vi "Untitled 2.vi"() -> ()   [LabVIEW 2017]
uses:
  <vilib>/Rock Robotics/SystemInterfaces/DIO/FPGA_DIOPWMChannel.ctl
  <vilib>/Rock Robotics/WPI/Joystick/WPI_JoystickDeviceEnum.ctl
  <vilib>/Rock Robotics/WPI/MotorControl/WPI_MotorControlOpen TalonSRX.vi
panel:
  in  "Output":dbl
  in  "stop":bool
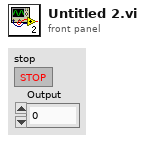
[diagram p1: front panel]
types:
  T1 = typedef "WPI_JoystickDeviceEnum.ctl" = enum16{"USB 0", "USB 1", "USB 2", "USB 3", "USB 4", "USB 5"}
  T2 = typedef "FPGA_DIOPWMChannel.ctl" = enum8{"PWM 0", "PWM 1", "PWM 2", "PWM 3", "PWM 4", "PWM 5", "PWM 6", "PWM 7", "PWM 8", "PWM 9", "PWM MXP 0", "PWM MXP 1", "PWM MXP 2", "PWM MXP 3", "PWM MXP 4", "PWM MXP 5", "PWM MXP 6", "PWM MXP 7", "PWM MXP 8", "PWM MXP 9", "Invalid"}
  T3 = typedef "WPI_MotorControlDeviceRef.ctl" = cluster{"DeviceStatus":errorcluster, "Type":T4, "PWM":cluster{"PWM Channel":T2, "DeadBand":T5}, "CAN":cluster{"Device Number":u8, "SetOutput VI Ref":variant, "GetOutput VI Ref":variant, "Enable VI Ref":variant, "Disable VI Ref":variant, "Data":variant}, "Invert":bool, "DIO PWM":cluster{"PWM \"Enable\" Channel":T2, "DIOChannel":T6, "PWM Rate":dbl}}
  T4 = typedef "WPI_MotorControlType.ctl" = enum16{"PWM", "CAN", "DIO PWM"}
  T5 = typedef "WPI_PWMDeadband.ctl" = cluster{"Name":string, "maxPositivePwm":i32, "minPositivePwm":i32, "centerPwm":i32, "maxNegativePwm":i32, "minNegativePwm":i32, "angularRange":u16}
  T6 = typedef "FPGA_DIOChannel.ctl" = enum8{"DIO 0", "DIO 1", "DIO 2", "DIO 3", "DIO 4", "DIO 5", "DIO 6", "DIO 7", "DIO 8", "DIO 9", "DIO MXP 0", "DIO MXP 1", "DIO MXP 2", "DIO MXP 3", "DIO MXP 4", "DIO MXP 5", "DIO MXP 6", "DIO MXP 7", "DIO MXP 8", "DIO MXP 9", "DIO MXP 10", "DIO MXP 11", "DIO MXP 12", "DIO MXP 13", "DIO MXP 14", "DIO MXP 15", "SPI Port CS1", "SPI Port CS2", "SPI Port CS3", "SPI Port MISO", "SPI Port MOSI", "Invalid"}
  T7 = typedef "WPI_JoystickDevRef.ctl" = cluster{"Device":T1}
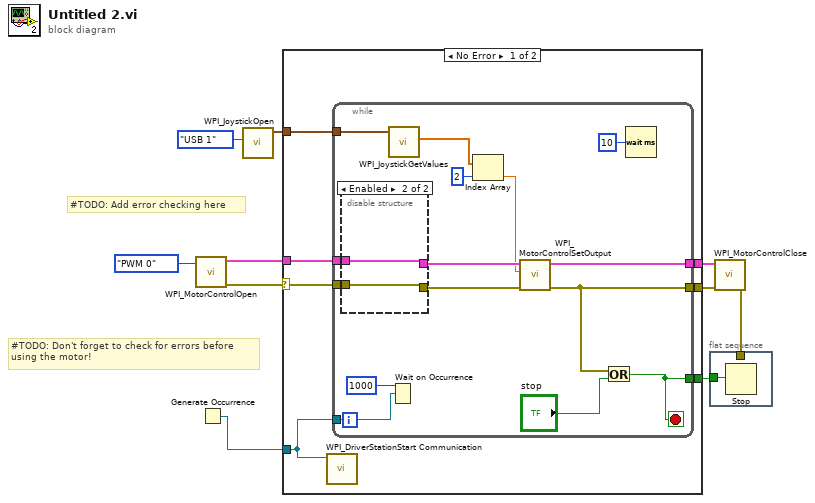
[diagram p0: block diagram]
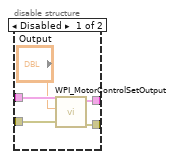
[diagram p2: hidden frame]
diagram:
  # "#TODO: Add error checking here"
  # "#TODO: Don't forget to check for errors before\nusing the motor!"
  n1 = call-poly <vilib>:"WPI_MotorControlOpen.vi"("PWM Channel"=FPGA_DIOPWMChannel."PWM 0") -> ("error out"=w1:errorcluster, "MotorControlDeviceRef"=w9:T3)  [unwired: 9 in]
  n2 = Generate Occurrence() -> (w5:refnum<k4>)
  n3 = call <vilib>:"WPI_JoystickOpen.vi"("JoystickDevice"=WPI_JoystickDeviceEnum."USB 1") -> ("JoystickDevRef"=w3:T7)  [unwired: 10 in]
  n4 = case shown="No Error" w1 {
    selector: w1 -> [w11 w41]
    tunnel: w9 -> [w17 w40]
    tunnel: [w16 w40] -> w8
    tunnel: [w15 w41] -> w7
    tunnel: w5 -> [w14 _]
    tunnel: w3 -> [w13 _]
    tunnel: [w12 _] -> w2
    frame No Error {
      n5 = call <vilib>:"WPI_DriverStationStart Communication.vi"("occurrence"=w14) -> ()  [unwired: 11 in]
      n6 = while {
        tunnel: w17 -> [w32]
        tunnel: w11 -> [w31]
        tunnel: [w22] -> w16
        tunnel: [w20] -> w15
        tunnel: w14 -> [w29]
        tunnel: w13 -> [w27]
        tunnel: [w18] -> w12
        stop <- w18 stop-if-true
        n7 = disable-structure shown="Enabled" {
          disable-tunnel: w32 -> [w37 w39]
          disable-tunnel: w31 -> [w36 w38]
          disable-tunnel: [w34 w39] -> w24
          disable-tunnel: [w33 w38] -> w23
          frame Disabled {
            n8 = call <vilib>:"WPI_MotorControlSetOutput.vi"("error in (no error)"=w36, "Output"="Output", "MotorControlDevRef"=w37) -> ("error out"=w33:errorcluster, "MotorControlDevRef"=w34:T3)  [unwired: 6 in, 1 out]
          }
          frame Enabled {
          }
        }
        n9 = Wait on Occurrence(2:w29, 3:1000 ("ms timeout (-1)")) -> ()  [unwired: 1 in, 1 out]
        n10 = call <vilib>:"WPI_JoystickGetValues.vi"("JoystickDevRef"=w27) -> ("Axes"=w25:dbl[])  [unwired: 6 in, 4 out]
        n11 = Index Array(array=w25, index=2) -> (element=w21:dbl)
        n12 = call <vilib>:"WPI_MotorControlSetOutput.vi"("error in (no error)"=w23, "Output"=w21, "MotorControlDevRef"=w24) -> ("error out"=w20:errorcluster, "MotorControlDevRef"=w22:T3)  [unwired: 6 in, 1 out]
        n13 = Or(x=w20, y="stop") -> (x .or. y?=w18:bool)
        n14 = Wait (ms)(milliseconds to wait=u32 10) -> ()  [unwired: 1 out]
      }
    }
    frame Error {
      # "#TODO: Add feedback to UI of error?\nLog or something..."
    }
  }
  n15 = flat-sequence {
    tunnel: w2 -> [w42]
    tunnel: w6 -> [_]
    frame #0 {
      n16 = Stop(stop? (T)=w42) -> ()
    }
  }
  n17 = call <vilib>:"WPI_MotorControlClose.vi"("error in"=w7, "MotorControlDevRef"=w8) -> ("error out"=w6:errorcluster)  [unwired: 9 in]
